vi "Discriminator Mode.vi"(7 "Read Value? (F)":bool, 8 "error in (no error)":errorcluster, 9 "Discriminator Mode (Fixed)":T1, 10 "Counter (A)":T2, 11 "VISA resource name":refnum<visa-resource-name>) -> (0 "error out":errorcluster, 1 "Discriminator Mode":T1, 3 "VISA resource name out":refnum<visa-resource-name>)   [LabVIEW 2013, in "SRS SR400.lvlib"]
doc: "<B>DM i { ,j }</B>\n\nThe DM command sets and reads the discriminator modes. i = 0,1, or 2 designates discriminator A,B, or T and is required. If j is included, the selected discriminator is set to FIXED, j=0, or SCAN, j=1. If j is absent, the mode of discriminator i is returned. The mode may be changed during a scan. If it is changed to SCAN, the level begins scanning from the start value on the next count period. If it is changed to FIXED, the level returns to the start value immediately."
uses:
  <instrlib>/SRS SR400/SRS SR400.lvlib
  <instrlib>/SRS SR400/Public/Typedefs/Counter.ctl
  <instrlib>/SRS SR400/Public/Typedefs/Discriminator Mode.ctl
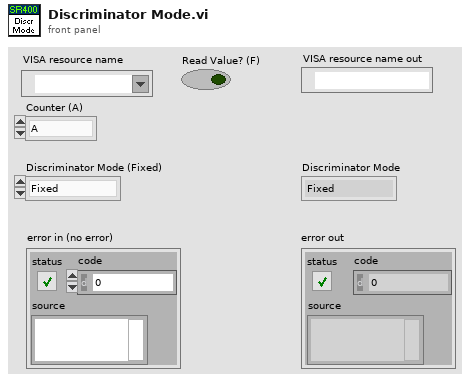
[diagram p1: front panel]
types:
  T1 = typedef "SRS SR400.lvlib/Discriminator Mode.ctl" = enum16{"Fixed", "Scan"}
  T2 = typedef "SRS SR400.lvlib/Counter.ctl" = enum16{"A", "B", "T"}
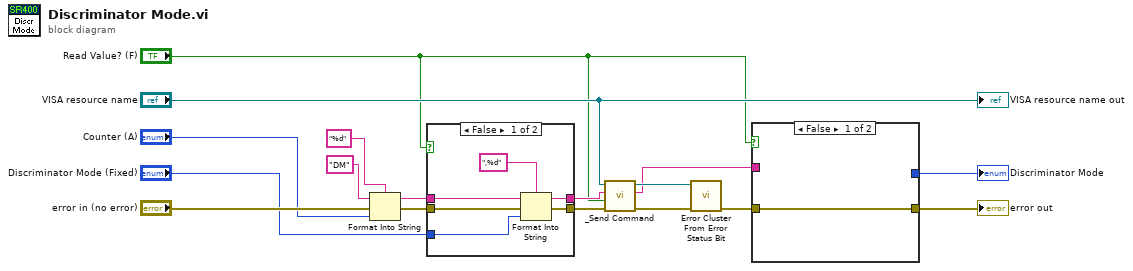
[diagram p0: block diagram]
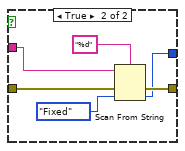
[diagram p2: hidden frame]
diagram:
  n1 = Format Into String(format string="%d", initial string="DM" ("command"), error in="error in (no error)", "Counter (A)") -> (resulting string=w15:string, error out=w16:errorcluster)
  n2 = case shown="False" "Read Value? (F)" {
    tunnel: w16 -> [w23 w24]
    tunnel: w15 -> [w18 w25]
    tunnel: [w21 w25] -> w12
    tunnel: [w20 w24] -> w11
    tunnel: "Discriminator Mode (Fixed)" -> [w19 _]
    frame False {
      n3 = Format Into String(format string=",%d", initial string=w18, error in=w23, w19) -> (resulting string=w21:string, error out=w20:errorcluster)
    }
    frame True {
    }
  }
  n4 = call <instrlib>:"_Send Command.vi"("error in (no error)"=w11, "Read Value? (F)"="Read Value? (F)", "Command"=w12, "VISA resource name"="VISA resource name") -> ("error out"=w6:errorcluster, "Response"=w4:string, "VISA resource name out"=w7:refnum<visa-resource-name>)  [unwired: 5 out]
  n5 = call <instrlib>:"Error Cluster From Error Status Bit.vi"("error in (no error)"=w6, "VISA resource name"=w7) -> ("error out"=w5:errorcluster)  [unwired: 8 in, 1 out]
  n6 = case shown="False" "Read Value? (F)" {
    tunnel: w5 -> [w26 w32]
    tunnel: w4 -> [_ w27]
    tunnel: [w26 w31] -> w2
    tunnel: [_ w28] -> w1
    frame False {
    }
    frame True {
      n7 = Scan From String(format string="%d", input string=w27, error in=w32, default 1=Discriminator_Mode."Fixed" ("Discriminator Mode (Fixed)")) -> (error out=w31:errorcluster, output 1=w28:T1)  [unwired: 1 in, 2 out]
    }
  }
  "error out" <- w2
  "Discriminator Mode" <- w1
  "VISA resource name out" <- "VISA resource name"
